vi "Write Average.vi"(10 "Average":cluster{"Count":u32, "On":bool}, 11 "Spectrum Analyzer in":refnum<class "Spectrum Analyzer.lvclass">) -> (3 "Spectrum Analyzer out":refnum<class "Spectrum Analyzer.lvclass">)   [LabVIEW 2020, in "Spectrum Analyzer.lvclass"]
uses:
  Spectrum Analyzer.lvclass
  Spectrum Analyzer.lvclass/Spectrum Analyzer.ctl
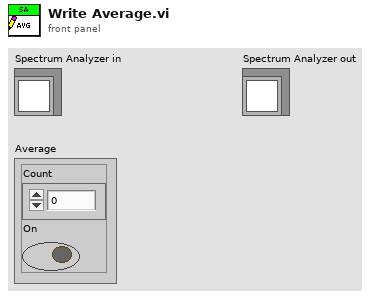
[diagram p1: front panel]
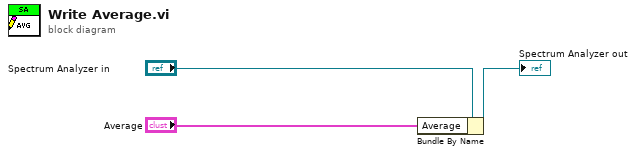
[diagram p0: block diagram]
diagram:
  n1 = Bundle By Name(cluster="Spectrum Analyzer in", "Average"="Average") -> (→"Spectrum Analyzer out":refnum<class "Spectrum Analyzer.lvclass">)
